vi "Restore Memento.vi"(8 "error in (no error)":errorcluster, 10 "Numeric Memento":refnum<class>, 11 "IMementoNumeric in":refnum<class "IMementoNumeric.lvclass">) -> (0 "error out":errorcluster, 3 "IMementoNumeric out":refnum<class "IMementoNumeric.lvclass">)   [LabVIEW 2009, in "IMementoNumeric.lvclass"]
uses:
  IMementoNumeric.lvclass
  MementoNumeric/MementoNumeric.lvclass
  Numeric Test Object.lvclass
  Source/IUnknown Class/IUnknown.lvclass
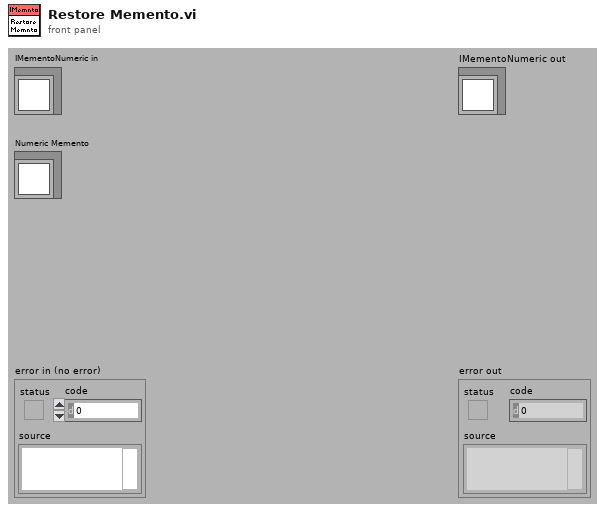
[diagram p1: front panel]
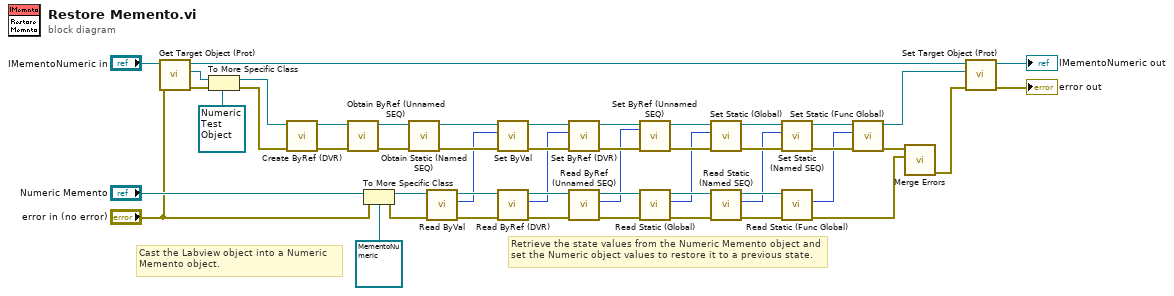
[diagram p0: block diagram]
diagram:
  # "Retrieve the state values from the Numeric Memento object and set the Numeric object values to restore it to a previous state."
  # "Cast the Labview object into a Numeric Memento object."
  n1 = call "Get Target Object (Prot).vi"("error in (no error)"="error in (no error)", "IUnknown in"="IMementoNumeric in") -> ("error out"=w4:errorcluster, "Target Object"=w5:refnum<class "Interfaceable.lvclass">, "IUnknown out"=w7:refnum<class "IMementoNumeric.lvclass">)  [unwired: 7 in]
  n2 = To More Specific Class(target class=refnum<class "Numeric Test Object.lvclass"> refnum ("Numeric"), reference=w5, error in=w4) -> (specific class reference=w1:refnum<class "Numeric Test Object.lvclass">, error out=w2:errorcluster)
  n3 = call-dynamic "Create ByRef (DVR).vi"("error in (no error)"=w2, "Numeric in"=w1) -> ("error out"=w28:errorcluster, "Numeric out"=w36:refnum<class "Numeric Test Object.lvclass">)  [unwired: 8 in]
  n4 = call-dynamic "Obtain ByRef (Unnamed SEQ).vi"("error in (no error)"=w28, "Numeric in"=w36) -> ("error out"=w27:errorcluster, "Numeric out"=w35:refnum<class "Numeric Test Object.lvclass">)  [unwired: 8 in]
  n5 = To More Specific Class(target class=refnum<class "MementoNumeric.lvclass"> refnum ("MementoNumeric"), reference="Numeric Memento", error in="error in (no error)") -> (specific class reference=w42:refnum<class "MementoNumeric.lvclass">, error out=w43:errorcluster)
  n6 = call-dynamic "Obtain Static (Named SEQ).vi"("error in (no error)"=w27, "Numeric in"=w35) -> ("error out"=w26:errorcluster, "Numeric out"=w34:refnum<class "Numeric Test Object.lvclass">)  [unwired: 8 in]
  n7 = call "Read ByVal.vi"("error in (no error)"=w43, "MementoNumeric in"=w42) -> ("error out"=w41:errorcluster, "ByVal"=w20:i32, "MementoNumeric out"=w50:refnum<class "MementoNumeric.lvclass">)  [unwired: 7 in]
  n8 = call-dynamic "Set ByVal.vi"("error in (no error)"=w26, "Int"=w20, "Numeric in"=w34) -> ("error out"=w25:errorcluster, "Numeric out"=w33:refnum<class "Numeric Test Object.lvclass">)  [unwired: 7 in]
  n9 = call "Read ByRef (DVR).vi"("error in (no error)"=w41, "MementoNumeric in"=w50) -> ("error out"=w40:errorcluster, "ByRef (DVR)"=w19:i32, "MementoNumeric out"=w49:refnum<class "MementoNumeric.lvclass">)  [unwired: 7 in]
  n10 = call-dynamic "Set ByRef (DVR).vi"("error in (no error)"=w25, "Int"=w19, "Numeric in"=w33) -> ("error out"=w24:errorcluster, "Numeric out"=w32:refnum<class "Numeric Test Object.lvclass">)  [unwired: 7 in]
  n11 = call "Read ByRef (Unnamed SEQ).vi"("error in (no error)"=w40, "MementoNumeric in"=w49) -> ("error out"=w39:errorcluster, "ByRef (Unnamed SEQ)"=w18:i32, "MementoNumeric out"=w48:refnum<class "MementoNumeric.lvclass">)  [unwired: 7 in]
  n12 = call-dynamic "Set ByRef (Unnamed SEQ).vi"("error in (no error)"=w24, "Int"=w18, "Numeric in"=w32) -> ("error out"=w23:errorcluster, "Numeric out"=w31:refnum<class "Numeric Test Object.lvclass">)  [unwired: 7 in]
  n13 = call "Read Static (Global).vi"("error in (no error)"=w39, "MementoNumeric in"=w48) -> ("error out"=w38:errorcluster, "Static (Global)"=w17:i32, "MementoNumeric out"=w47:refnum<class "MementoNumeric.lvclass">)  [unwired: 7 in]
  n14 = call-dynamic "Set Static (Global).vi"("error in (no error)"=w23, "Int"=w17, "Numeric in"=w31) -> ("error out"=w22:errorcluster, "Numeric out"=w30:refnum<class "Numeric Test Object.lvclass">)  [unwired: 7 in]
  n15 = call "Read Static (Named SEQ).vi"("error in (no error)"=w38, "MementoNumeric in"=w47) -> ("error out"=w37:errorcluster, "Static (Named SEQ)"=w16:i32, "MementoNumeric out"=w46:refnum<class "MementoNumeric.lvclass">)  [unwired: 7 in]
  n16 = call-dynamic "Set Static (Named SEQ).vi"("error in (no error)"=w22, "Int"=w16, "Numeric in"=w30) -> ("error out"=w21:errorcluster, "Numeric out"=w29:refnum<class "Numeric Test Object.lvclass">)  [unwired: 7 in]
  n17 = call "Read Static (Func Global).vi"("error in (no error)"=w37, "MementoNumeric in"=w46) -> ("error out"=w12:errorcluster, "Static (Func Global)"=w15:i32)  [unwired: 7 in, 1 out]
  n18 = call-dynamic "Set Static (Func Global).vi"("error in (no error)"=w21, "Int"=w15, "Numeric in"=w29) -> ("error out"=w13:errorcluster, "Numeric out"=w14:refnum<class "Numeric Test Object.lvclass">)  [unwired: 7 in]
  n19 = call <vilib>:"Merge Errors.vi"("error in 2 (no error)"=w12, "error in 1 (no error)"=w13) -> ("error out"=w11:errorcluster)  [unwired: 5 in]
  n20 = call "Set Target Object (Prot).vi"("error in (no error)"=w11, "Target Object"=w14, "IUnknown in"=w7) -> ("error out"=→"error out":errorcluster, "IUnknown out"=→"IMementoNumeric out":refnum<class "IMementoNumeric.lvclass">)  [unwired: 7 in]
